vi "NI-XNET Monitor Get Comm State.vi"(8 "Error In":errorcluster, 11 "Process  Data In":T1) -> (0 "Error Out":errorcluster, 3 "Process  Data Out":T1)   [LabVIEW 2017, in "NI-XNET Monitor Engine.lvlib"]
uses:
  NI-XNET Monitor Engine.lvlib
  RTMonitorRefnums.ctl
  <vilib>/NI/NIVS Inline Async API/_Data Access Engine/Data Access Engine/Types/Write.DVR.ctl
  <vilib>/NI/NIVS Inline Async API/_Data Access Engine/Access Type Classes/Write/Write.lvclass
  <vilib>/NI/NIVS Inline Async API/_Data Access Engine/Access Type Classes/Write/Write.lvclass/Write.ctl
  <vilib>/NI/NIVS Inline Async API/_Data Access Engine/Data Access Engine/Methods/Write.Data.vi
  <vilib>/NI/NIVS Inline Async API/_Data Access Engine/Access Type Classes/Write/Write.ProcessData.vi
  <vilib>/xnet/xnet.llb/XNET Read (State CAN Comm).vi
  <vilib>/xnet/xnet.llb/XNET Read (State FlexRay Comm).vi
  <vilib>/xnet/xnet.llb/XNET Read (State LIN Comm).vi
  <vilib>/NI/NIVS Inline Async API/_Data Access Engine/Data Access Engine/Data Access Engine.lvclass
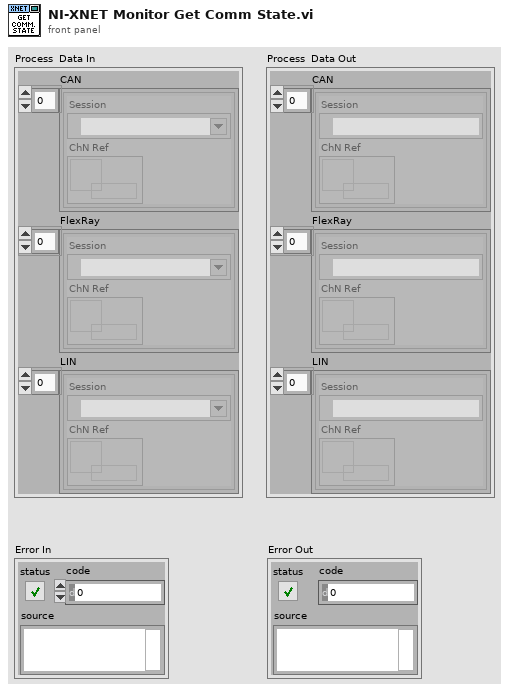
[diagram p1: front panel]
types:
  T1 = typedef "NI-XNET Monitor Engine.lvlib/RTMonitorRefnums.ctl" = cluster{"CAN":cluster{"Session":refnum<k21>, "ChN Ref":T2}[], "FlexRay":cluster{"Session":refnum<k21>, "ChN Ref":T2}[], "LIN":cluster{"Session":refnum<k21>, "ChN Ref":T2}[]}
  T2 = typedef "Data Access Engine.lvlib/Data Access Engine.lvclass/Write.DVR.ctl" = refnum<data-value>
  T3 = typedef "XNET CAN Comm.ctl" = cluster{"fault code":i32, "fault?":bool, "communication state":T4, "last error":T5, "receive error counter":u8, "transmit error counter":u8, "transceiver error?":bool, "sleep?":bool}
  T4 = typedef "XNET CAN Comm State.ctl" = u8
  T5 = typedef "XNET CAN Last Err.ctl" = u8
  T6 = typedef "XNET FlexRay Comm.ctl" = cluster{"fault code":i32, "fault?":bool, "FlexRay POC state":T7, "clock correction failed":u8, "passive to active count":u8, "channel A sleep?":bool, "channel B sleep?":bool}
  T7 = typedef "XNET FlexRay POC State.ctl" = u8
  T8 = typedef "XNET LIN Comm.ctl" = cluster{"fault code":i32, "fault?":bool, "communication state":T9, "last error":T10, "last error received":u8, "last error expected":u8, "last error identifier":u8, "sleep?":bool, "transceiver ready?":bool, "schedule index":u8}
  T9 = typedef "XNET LIN Comm State.ctl" = u8
  T10 = typedef "XNET LIN Last Err.ctl" = u8
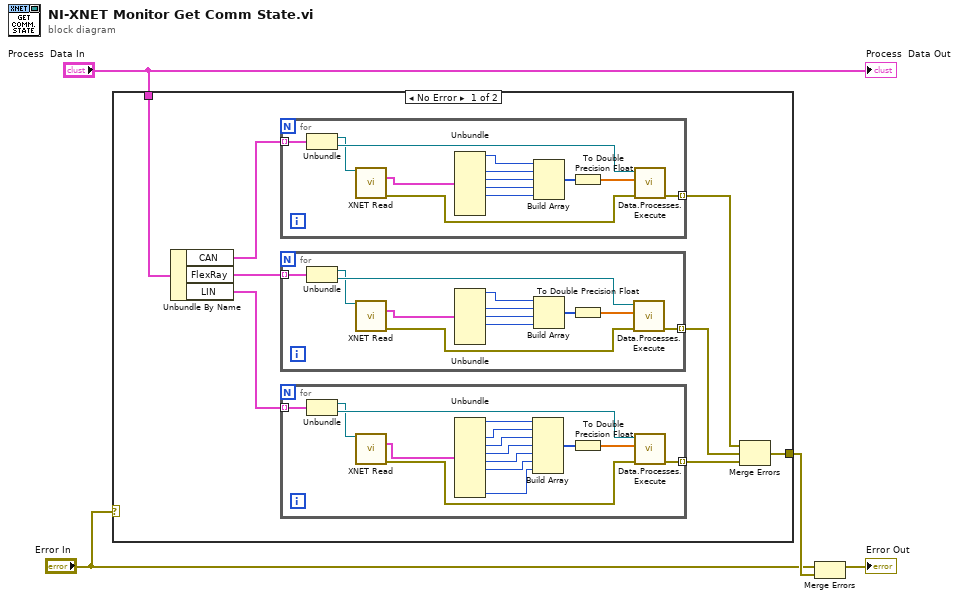
[diagram p0: block diagram]
diagram:
  n1 = case shown="No Error" "Error In" {
    tunnel: "Process  Data In" -> [w12 _]
    tunnel: [w5 _] -> w2
    frame No Error {
      n2 = Unbundle By Name(w12) -> ("CAN"=w11:cluster{"Session":refnum<k21>, "ChN Ref":T2}[], "FlexRay"=w10:cluster{"Session":refnum<k21>, "ChN Ref":T2}[], "LIN"=w6:cluster{"Session":refnum<k21>, "ChN Ref":T2}[])
      n3 = for {
        tunnel: w11 -> [w52] mode=indexing
        tunnel: [w49] -> w7 mode=indexing
        n4 = Unbundle(w52) -> ("Session"=w46:refnum<k21>, "ChN Ref"=w47:T2)
        n5 = call-poly <vilib>:"XNET Read.vi"("session in"=w46) -> ("CAN comm"=w48:T3, "error out"=w50:errorcluster)  [unwired: 12 in, 1 out]
        n6 = Unbundle(w48) -> ("fault code"=w41:i32, "communication state"=w45:T4, "last error"=w44:T5, "receive error counter"=w43:u8, "transmit error counter"=w42:u8)  [unwired: 3 out]
        n7 = Build Array(w41, w45, w44, w43, w42) -> (w51:i32[])
        n8 = To Double Precision Float(number=w51) -> (double precision float=w40:dbl[])
        n9 = call-poly <vilib>:"Data.Processes.Execute.vi"("error in (no error)"=w50, "Values"=w40, "Ref"=w47) -> ("error out"=w49:errorcluster)  [unwired: 8 in]
      }
      n10 = for {
        tunnel: w10 -> [w39] mode=indexing
        tunnel: [w35] -> w8 mode=indexing
        n11 = Unbundle(w39) -> ("Session"=w33:refnum<k21>, "ChN Ref"=w34:T2)
        n12 = call-poly <vilib>:"XNET Read.vi"("session in"=w33) -> ("FlexRay comm"=w38:T6, "error out"=w29:errorcluster)  [unwired: 12 in, 1 out]
        n13 = Unbundle(w38) -> ("fault code"=w37:i32, "FlexRay POC state"=w32:T7, "clock correction failed"=w31:u8, "passive to active count"=w30:u8)  [unwired: 3 out]
        n14 = Build Array(w37, w32, w31, w30) -> (w36:i32[])
        n15 = To Double Precision Float(number=w36) -> (double precision float=w28:dbl[])
        n16 = call-poly <vilib>:"Data.Processes.Execute.vi"("error in (no error)"=w29, "Values"=w28, "Ref"=w34) -> ("error out"=w35:errorcluster)  [unwired: 8 in]
      }
      n17 = for {
        tunnel: w6 -> [w27] mode=indexing
        tunnel: [w23] -> w9 mode=indexing
        n18 = Unbundle(w27) -> ("Session"=w20:refnum<k21>, "ChN Ref"=w21:T2)
        n19 = call-poly <vilib>:"XNET Read.vi"("session in"=w20) -> ("LIN comm"=w26:T8, "error out"=w22:errorcluster)  [unwired: 12 in, 1 out]
        n20 = Unbundle(w26) -> ("fault code"=w25:i32, "communication state"=w19:T9, "last error"=w18:T10, "last error received"=w17:u8, "last error expected"=w16:u8, "last error identifier"=w15:u8, "schedule index"=w14:u8)  [unwired: 3 out]
        n21 = Build Array(w25, w19, w18, w17, w16, w15, w14) -> (w24:i32[])
        n22 = To Double Precision Float(number=w24) -> (double precision float=w13:dbl[])
        n23 = call-poly <vilib>:"Data.Processes.Execute.vi"("error in (no error)"=w22, "Values"=w13, "Ref"=w21) -> ("error out"=w23:errorcluster)  [unwired: 8 in]
      }
      n24 = Merge Errors(w7, w8, w9) -> (w5:errorcluster)
    }
    frame Error {
    }
  }
  n25 = Merge Errors("Error In", w2) -> (→"Error Out":errorcluster)
  "Process  Data Out" <- "Process  Data In"
